vi "Explorer_ReadConsole.vi"(8 "index in":i32, 11 "String in":refnum<vi>) -> (0 "index out":i32, 1 "New Line":string, 2 "New point?":bool, 3 "String out":refnum<vi>)   [LabVIEW 2020]
panel:
  out "Value":string
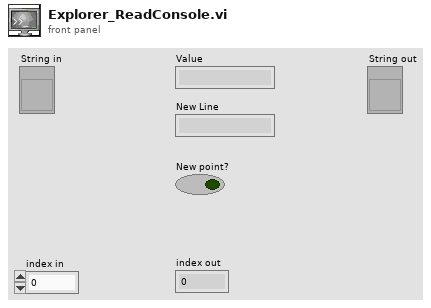
[diagram p1: front panel]
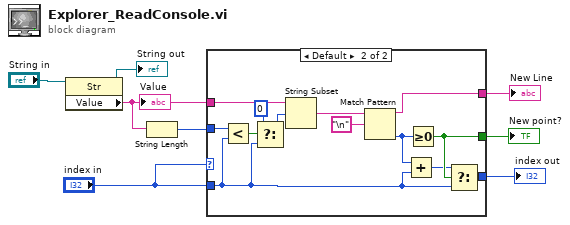
[diagram p0: block diagram]
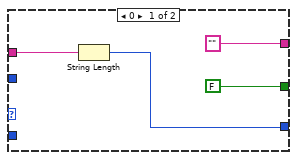
[diagram p2: hidden frame]
diagram:
  n1 = property class="Str"(reference="String in") -> (reference out=→"String out":refnum<vi>, "Value"=w2:string)  [unwired: 1 in, 1 out]
  "Value" <- w2
  n2 = String Length(string=w2) -> (length=w1:i32)
  n3 = case shown="Default" "index in" {
    tunnel: [FALSE w25] -> w8
    tunnel: "index in" -> [_ w14]
    tunnel: [w9 w22] -> w7
    tunnel: w2 -> [w10 w19]
    tunnel: ["" ("Value") w18] -> w5
    tunnel: w1 -> [_ w17]
    frame 0 {
      n4 = String Length(string=w10) -> (length=w9:i32)
    }
    frame Default {
      n5 = Less?(x=w17, y=w14) -> (x < y?=w16:bool)
      n6 = Select(t=0, s=w16, f=w14) -> (s? t:f=w13:i32)
      n7 = String Subset(string=w19, offset (0)=w13) -> (substring=w20:string)  [unwired: 1 in]
      n8 = Match Pattern(string=w20, regular expression="\n") -> (before substring=w18:string, offset past match=w23:i32)  [unwired: 1 in, 2 out]
      n9 = Add(x=w23, y=w14) -> (x+y=w24:i32)
      n10 = Greater Or Equal To 0?(x=w23) -> (x >= 0?=w25:bool)
      n11 = Select(t=w24, s=w25, f=w14) -> (s? t:f=w22:i32)
    }
  }
  "New point?" <- w8
  "index out" <- w7
  "New Line" <- w5
